vi "read MagspecCameraLineouts.vi"(11 "File Path":path) -> (3 "calib":T1)   [LabVIEW 2013, in "MagSpecStitcher.lvclass"]
uses:
  MagSpecStitcher.lvclass
  LineoutStats.ctl
  Read From Spreadsheet File (DBL).vi
panel:
  out "momentum":dbl[](array[numeric])
  out "Spectrum lineout path":path
  out "all rows":dbl[][](array[numeric]) format="%0.3f"
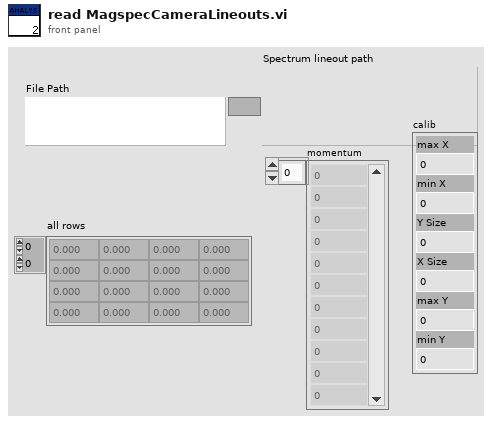
[diagram p1: front panel]
types:
  T1 = typedef "LineoutStats.ctl" = cluster{"max X":dbl, "min X":dbl, "Y Size":dbl, "X Size":dbl, "max Y":dbl, "min Y":dbl}
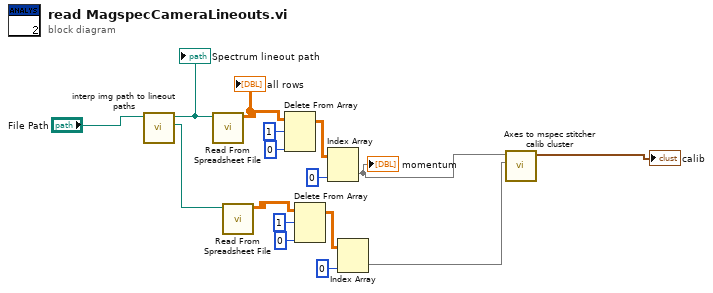
[diagram p0: block diagram]
diagram:
  n1 = call "interp img path to lineout paths.vi"("Interp image path"="File Path") -> ("angle lineout path"=w4:path, "Spectrum lineout path"=w15:path)  [unwired: 8 in, 1 out]
  "Spectrum lineout path" <- w15
  n2 = call-poly "Read From Spreadsheet File.vi"("file path (dialog if empty)"=w15) -> ("all rows"=w13:dbl[][])  [unwired: 6 in, 4 out]
  "all rows" <- w13
  n3 = call-poly "Read From Spreadsheet File.vi"("file path (dialog if empty)"=w4) -> ("all rows"=w6:dbl[][])  [unwired: 6 in, 4 out]
  n4 = Delete From Array(array=w13, length=1, index (row)=0) -> (array with subset deleted=w12:dbl[][])  [unwired: 1 in, 1 out]
  n5 = Delete From Array(array=w6, length=1, index (row)=0) -> (array with subset deleted=w7:dbl[][])  [unwired: 1 in, 1 out]
  n6 = Index Array(array=w12, index (col)=0 ("disabled index (col)")) -> (element=w1:dbl[])  [unwired: 1 in]
  "momentum" <- w1
  n7 = Index Array(array=w7, index (col)=0 ("disabled index (col)")) -> (element=w3:dbl[])  [unwired: 1 in]
  n8 = call "Axes to mspec stitcher calib cluster.vi"("Angle axis"=w3, "Energy axis"=w1) -> ("calib"=→"calib":T1)  [unwired: 9 in]
